vi "阀口名称设置.vi"() -> ()   [LabVIEW 2016, in "斯坦道总磷.lvlib"]
panel:
  in  "取消":bool
  in  "确认":bool
  in  "阀口名称":T1={"V"="试剂1", "V 2"="试剂2", "V 3"="试剂3", "V 4"="试剂4", "V 5"="试剂5", "V 6"="试剂6", "V 7"="试剂7", "V 8"="试剂8", "V 9"="试剂9", "V 10"="试剂10", "V 11"="试剂11", "V 12"="试剂12", "V9-1"="试剂13", "V9-2"="试剂14"}
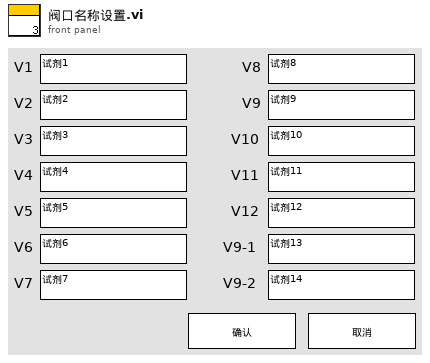
[diagram p1: front panel]
types:
  T1 = cluster{"V":string, "V 2":string, "V 3":string, "V 4":string, "V 5":string, "V 6":string, "V 7":string, "V 8":string, "V 9":string, "V 10":string, "V 11":string, "V 12":string, "V9-1":string, "V9-2":string}
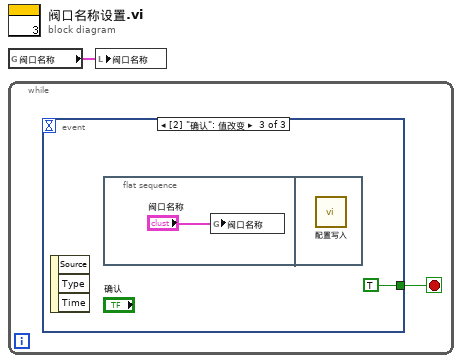
[diagram p0: block diagram]
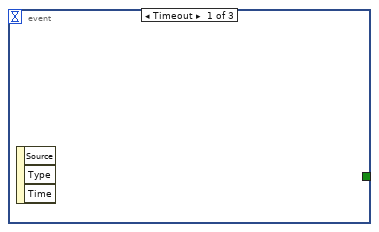
[diagram p2: hidden frame]
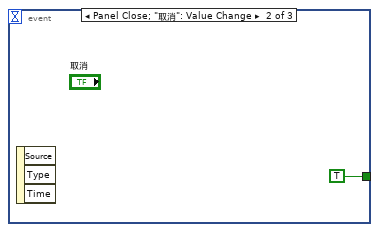
[diagram p3: hidden frame]
diagram:
  n1 = global read "总磷总氮断电保存全局变量.vi" "阀口名称"() -> (w1:T1)
  n2 = while {
    stop <- w2 stop-if-true
    n3 = event shown="[2] \"确认\": 值改变" {
      selector: _ -> [_ _ _]
      dyn-events: _ -> [_ _ _]
      timeout: _ -> [_ _ _]
      tunnel: [_ TRUE TRUE] -> w2
      event Timeout {
        n4 = event-data() -> ()  [unwired: 1 in, 3 out]
      }
      event Panel Close; "取消": Value Change {
        n5 = event-data() -> ()  [unwired: 1 in, 3 out]
      }
      event "确认": Value Change {
        n6 = event-data() -> ()  [unwired: 1 in, 3 out]
        n7 = flat-sequence {
          frame #0 {
            n8 = global write "总磷总氮断电保存全局变量.vi" "阀口名称"("阀口名称") -> ()
          }
          frame #1 {
            n9 = call "配置写入.vi"() -> ()  [unwired: 11 in, 1 out]
          }
        }
      }
    }
  }
  n10 = local write "阀口名称"(w1) -> ()
